vi "Update Tree for Candidate Info.vi"(0 "Tree Ref":refnum<vi>, 5 "Candidates":T1[](array[typedef]), 11 "error in (no error)":errorcluster) -> (15 "error out":errorcluster)   [LabVIEW 2014, in "Coding Platform.lvlib"]
uses:
  Coding Platform.lvlib
  Typedefs/Candidate.ctl
  Typedefs/Candidate State.ctl
  Typedefs/Answer Info.ctl
  Typedefs/Answer State.ctl
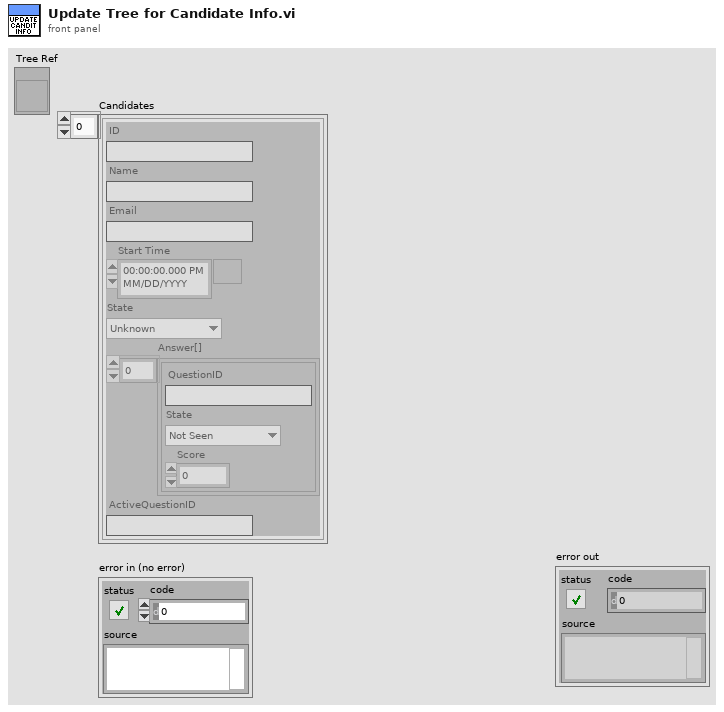
[diagram p1: front panel]
types:
  T1 = typedef "Coding Platform.lvlib/Candidate.ctl" = cluster{"ID":string, "Name":string, "Email":string, "Start Time":timestamp, "State":T2, "Answer[]":T3[], "ActiveQuestionID":string}
  T2 = typedef "Coding Platform.lvlib/Candidate State.ctl" = enum16{"Unknown", "LoggedIn", "In Test", "Completed Test"}
  T3 = typedef "Coding Platform.lvlib/Answer Info.ctl" = cluster{"QuestionID":string, "State":T4, "Score":u64}
  T4 = typedef "Coding Platform.lvlib/Answer State.ctl" = enum16{"Not Seen", "In Progress", "Completed"}
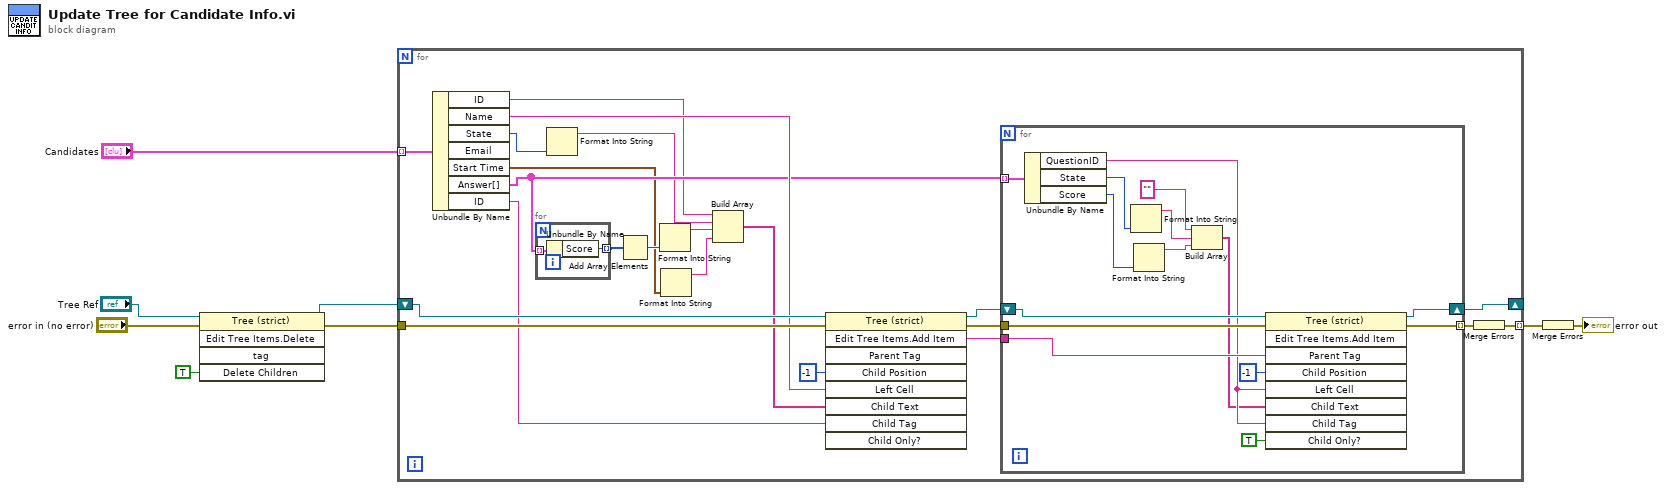
[diagram p0: block diagram]
diagram:
  n1 = invoke class="Tree (strict)" method="Edit Tree Items.Delete"(reference="Tree Ref", error in="error in (no error)", "Delete Children"=TRUE ("Delete Children?")) -> (reference out=w2:refnum<vi>, error out=w4:errorcluster)  [unwired: 2 in, 3 out]
  n2 = for {
    tunnel: "Candidates" -> [w30] mode=indexing
    shift-right: [w24] -> _
    shift-left: w2 -> [w25]
    tunnel: [w27] -> w7 mode=indexing
    tunnel: w4 -> [w28]
    n3 = Unbundle By Name(w30) -> ("ID"=w17:string, "Name"=w21:string, "State"=w16:T2, "Start Time"=w11:timestamp, "Answer[]"=w19:T3[], "ID"=w20:string)  [unwired: 1 out]
    n4 = for {
      tunnel: w19 -> [w32] mode=indexing
      tunnel: [w31] -> w18 mode=indexing
      n5 = Unbundle By Name(w32) -> ("Score"=w31:u64)
    }
    n6 = Format Into String(w16) -> (resulting string=w15:string)  [unwired: 3 in, 1 out]
    n7 = Add Array Elements(numeric array=w18) -> (sum=w13:u64)
    n8 = Format Into String(w13) -> (resulting string=w14:string)  [unwired: 3 in, 1 out]
    n9 = Format Into String(w11) -> (resulting string=w10:string)  [unwired: 3 in, 1 out]
    n10 = Build Array(w17, w15, w14, w10) -> (w12:string[])
    n11 = invoke class="Tree (strict)" method="Edit Tree Items.Add Item"(reference=w25, error in=w28, "Child Position"=-1, "Left Cell"=w21, "Child Text"=w12, "Child Tag"=w20) -> (reference out=w23:refnum<vi>, error out=w26:errorcluster, "Edit Tree Items:Add Item"=w22:string)  [unwired: 3 in, 6 out]
    n12 = for {
      tunnel: w19 -> [w47] mode=indexing
      tunnel: [w45] -> w29 mode=indexing
      tunnel: w26 -> [w46]
      shift-right: [w43] -> w24
      shift-left: w23 -> [w44]
      tunnel: w22 -> [w42]
      n13 = Unbundle By Name(w47) -> ("QuestionID"=w41:string, "State"=w40:T4, "Score"=w39:u64)
      n14 = Format Into String(w40) -> (resulting string=w37:string)  [unwired: 3 in, 1 out]
      n15 = Format Into String(w39) -> (resulting string=w38:string)  [unwired: 3 in, 1 out]
      n16 = Build Array("" ("element"), w37, w38) -> (w35:string[])
      n17 = invoke class="Tree (strict)" method="Edit Tree Items.Add Item"(reference=w44, error in=w46, "Parent Tag"=w42, "Child Position"=-1, "Left Cell"=w41, "Child Text"=w35, "Child Tag"=w41, "Child Only?"=TRUE) -> (reference out=w43:refnum<vi>, error out=w45:errorcluster)  [unwired: 1 in, 7 out]
    }
    n18 = Merge Errors(w29) -> (w27:errorcluster)
  }
  n19 = Merge Errors(w7) -> (→"error out":errorcluster)
